vi "Setup Channel 1 for measurement.vi"(0 "Session In":refnum<visa-resource-name>="GPIB0::16::INSTR", 5 "CF (Hz)":dbl=100000000.0, 7 "MKRx (Hz)":dbl=100000000.0, 11 "error in":errorcluster {"code" format="%.0x"}, 12 "RefLvl (dBm)":dbl=20.0, 13 "Attn Lvl (dB)":dbl=20.0) -> (4 "Session Out":refnum<visa-resource-name>, 15 "error out":errorcluster {"code" format="%.0x"})   [LabVIEW 2018]
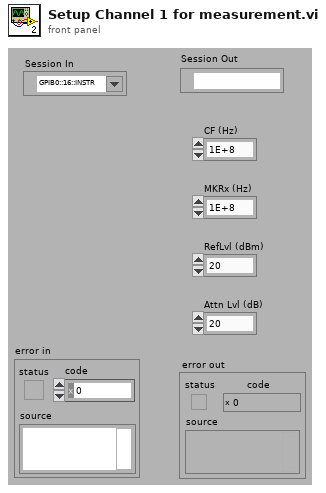
[diagram p1: front panel]
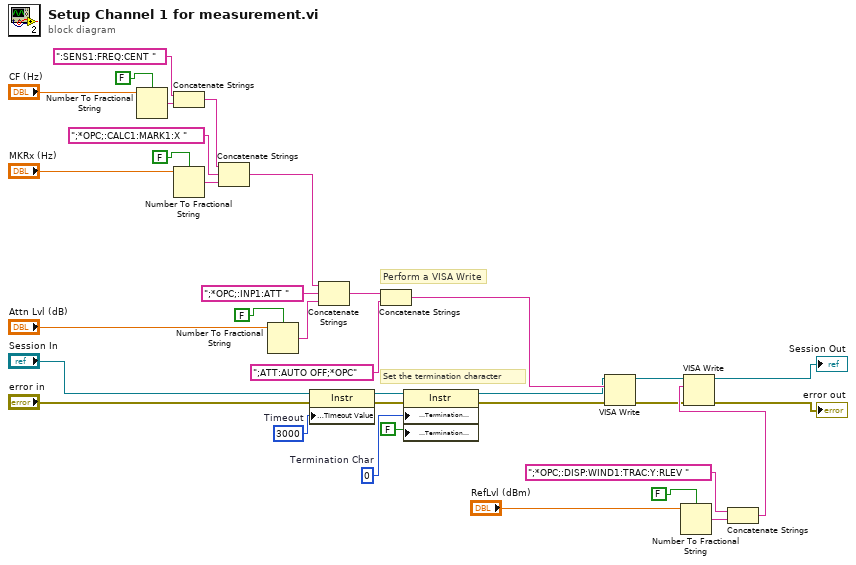
[diagram p0: block diagram]
diagram:
  w22 = u8 0  # Termination Char
  w26 = u32 3000  # Timeout
  # "Perform a VISA Write"
  # "Set the termination character"
  n1 = Number To Fractional String(use system decimal point (T)=FALSE, number="CF (Hz)") -> (F-format string=w19:string)  [unwired: 2 in]
  n2 = Concatenate Strings(":SENS1:FREQ:CENT " ("staticText"), w19) -> (w16:string)
  n3 = Number To Fractional String(use system decimal point (T)=FALSE, number="MKRx (Hz)") -> (F-format string=w17:string)  [unwired: 2 in]
  n4 = Concatenate Strings(w16, ";*OPC;:CALC1:MARK1:X " ("staticText"), w17) -> (w6:string)
  n5 = Number To Fractional String(use system decimal point (T)=FALSE, number="Attn Lvl (dB)") -> (F-format string=w12:string)  [unwired: 2 in]
  n6 = property class="Instr"(reference="Session In", error in="error in", "General Settings:Timeout Value"=w26) -> (reference out=w21:refnum<visa-resource-name>, error out=w24:errorcluster)
  n7 = Concatenate Strings(w6, ";*OPC;:INP1:ATT " ("staticText"), w12) -> (w9:string)
  n8 = Concatenate Strings(w9, ";ATT:AUTO OFF;*OPC" ("StaticText")) -> (w10:string)
  n9 = property class="Instr"(reference=w21, error in=w24, "Message Based Settings:Termination Character"=w22, "Message Based Settings:Termination Character Enable"=FALSE ("enable")) -> (reference out=w7:refnum<visa-resource-name>, error out=w23:errorcluster)
  n10 = VISA Write(VISA resource name=w7, write buffer=w10, error in (no error)=w23) -> (VISA resource name out=w4:refnum<visa-resource-name>, error out=w1:errorcluster)  [unwired: 1 out]
  n11 = Number To Fractional String(use system decimal point (T)=FALSE, number="RefLvl (dBm)") -> (F-format string=w14:string)  [unwired: 2 in]
  n12 = Concatenate Strings(";*OPC;:DISP:WIND1:TRAC:Y:RLEV " ("staticText"), w14) -> (w5:string)
  n13 = VISA Write(VISA resource name=w4, write buffer=w5, error in (no error)=w1) -> (VISA resource name out=→"Session Out":refnum<visa-resource-name>, error out=→"error out":errorcluster)  [unwired: 1 out]
